vi "ModeTranslate.vi"(11 "Status 2":u32) -> (3 "String":string)   [LabVIEW 2015]
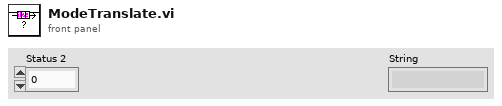
[diagram p1: front panel]
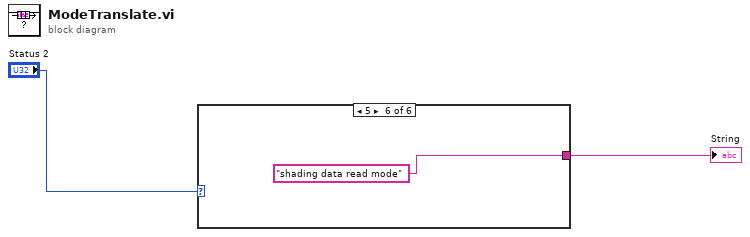
[diagram p0: block diagram]
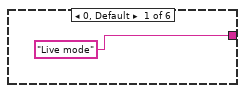
[diagram p2: hidden frame]
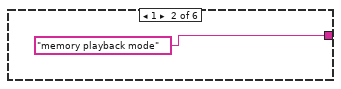
[diagram p3: hidden frame]
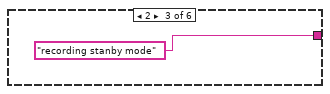
[diagram p4: hidden frame]
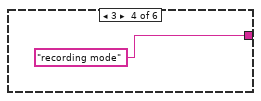
[diagram p5: hidden frame]
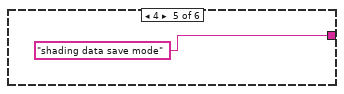
[diagram p6: hidden frame]
diagram:
  n1 = case shown="5" "Status 2" {
    tunnel: ["Live mode" ("String") "memory playback mode" ("String") "recording stanby mode" ("String") "recording mode" ("String") "shading data save mode" ("String") "shading data read mode" ("String")] -> w1
    frame 0, Default {
    }
    frame 1 {
    }
    frame 2 {
    }
    frame 3 {
    }
    frame 4 {
    }
    frame 5 {
    }
  }
  "String" <- w1
